vi "Default Contour Property.vi"(11 "Plot ID":i32) -> (3 "Default Property":T1={"General Property"={"Plot Name"="", "Coordinate System"=enum."Cartesian", "Opacity"=0.0}, "Projection Property"={"Draw XY"=FALSE, "Draw YZ"=FALSE, "Draw XZ"=FALSE}, "Plot Property"={"Line Style"=enum."None", "Line Width"=0.0, "Line Color"=0, "Antialiasing"=FALSE, "Color Ramp Cluster"={"Color Ramp Style"=enum."None", "Color Ramp Array"=[16711934, 393471, 57855, 4390754, 16449346, 16744722, 16711680], "Color Ramp Index"=[45, 91, 133, 175, 219, 255], "Interpolate?"=FALSE, "Logarithm?"=FALSE}}, "Contour Property"={"Contour Type"=enum."Contour with surface", "Axis Basis"=enum."Z-Axis", "Level List"=[], "Level Mode"=enum."Levels", "Levels"=0, "Interval"=0.0}})   [LabVIEW 2020, in "3D Contour.lvclass"]
uses:
  <vilib>/Math Plots/3D Math Plots/3D Contour/3D Contour/3D Contour.lvclass
  <vilib>/Math Plots/3D Math Plots/3D Contour/3D Contour/Typedef/3D Contour Property.ctl
  <vilib>/Math Plots/3D Math Plots/3D Plot/3D Plot/Typedef/Line Type.ctl
  <vilib>/Math Plots/3D Math Plots/3D Plot/3D Plot/Typedef/Color Ramp Cluster.ctl
  <vilib>/Math Plots/3D Math Plots/3D Plot/3D Plot/3D Plot.lvclass
panel:
  in  "Name Prefix":string="Plot "
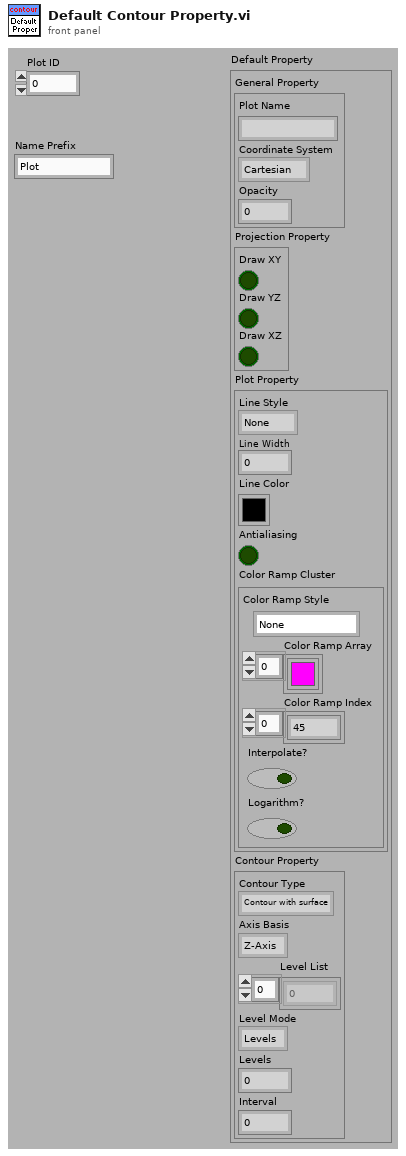
[diagram p1: front panel]
types:
  T1 = typedef "3D Contour.lvclass/3D Contour Property.ctl" = cluster{"General Property":cluster{"Plot Name":string, "Coordinate System":enum16{"Cartesian", "Cylindrical", "Spherical"}, "Opacity":sgl}, "Projection Property":cluster{"Draw XY":bool, "Draw YZ":bool, "Draw XZ":bool}, "Plot Property":cluster{"Line Style":T2, "Line Width":sgl, "Line Color":u32, "Antialiasing":bool, "Color Ramp Cluster":T3}, "Contour Property":cluster{"Contour Type":enum16{"Contour", "Contour with surface"}, "Axis Basis":enum16{"X-Axis", "Y-Axis", "Z-Axis"}, "Level List":sgl[], "Level Mode":enum16{"Levels", "Interval", "Level List"}, "Levels":u16, "Interval":sgl}}
  T2 = typedef "3D Plot.lvclass/Line Type.ctl" = enum16{"None", "Solid", "Dash", "Dot", "Dash Dot"}
  T3 = typedef "3D Plot.lvclass/Color Ramp Cluster.ctl" = cluster{"Color Ramp Style":enum16{"None", "Shaded", "Color spectrum", "Grey scale", "Custom"}, "Color Ramp Array":u32[], "Color Ramp Index":i32[], "Interpolate?":bool, "Logarithm?":bool}
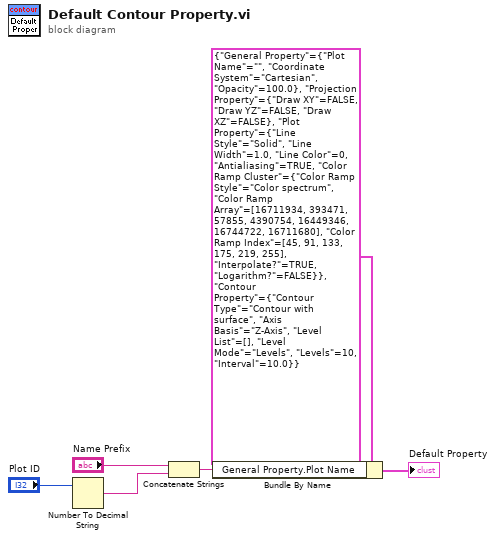
[diagram p0: block diagram]
diagram:
  n1 = Number To Decimal String(number="Plot ID") -> (decimal integer string=w6:string)  [unwired: 1 out]
  n2 = Concatenate Strings("Name Prefix", w6) -> (w3:string)
  n3 = Bundle By Name(cluster=T1 {"General Property"={"Plot Name"="", "Coordinate System"=enum."Cartesian", "Opacity"=100.0}, "Projection Property"={"Draw XY"=FALSE, "Draw YZ"=FALSE, "Draw XZ"=FALSE}, "Plot Property"={"Line Style"=enum."Solid", "Line Width"=1.0, "Line Color"=0, "Antialiasing"=TRUE, "Color Ramp Cluster"={"Color Ramp Style"=enum."Color spectrum", "Color Ramp Array"=[16711934, 393471, 57855, 4390754, 16449346, 16744722, 16711680], "Color Ramp Index"=[45, 91, 133, 175, 219, 255], "Interpolate?"=TRUE, "Logarithm?"=FALSE}}, "Contour Property"={"Contour Type"=enum."Contour with surface", "Axis Basis"=enum."Z-Axis", "Level List"=[], "Level Mode"=enum."Levels", "Levels"=10, "Interval"=10.0}} ("new element/subarray"), "General Property.Plot Name"=w3) -> (→"Default Property":T1)
